vi "Main.vi"() -> ()   [LabVIEW 2018]
doc: "This Continuous Measurement sample project is based on the Queued Message Handler template.\n\nThe Event Handling Loop generates messages based on user interface actions.\n\nThe Message Handling Loop processes messages generated by the Event Handling Loop, or by other messages. There are also Acquisition and Logging message handling loop subVIs, and a chart updating loop."
uses:
  Settings/Settings.ctl
  Acquisition/Hardware Configuration.ctl
  Logging/Logging Configuration.ctl
  controls/UI Data.ctl
  controls/UI State.ctl
  support/Message Queue/Enqueue Message (Single).vi
  support/Message Queue/Enqueue Message (Array).vi
  <vilib>/Utility/error.llb/Error Cluster From Error Code.vi
  <vilib>/ErrorRing/Error Ring.xnode
  Acquisition/Acquisition.lvlib
  Logging/Logging.lvlib
  Settings/Settings.lvlib
  support/User Event - Stop/User Event - Stop.lvlib
  support/Message Queue/Message Queue.lvlib
  Settings/Settings Dialog.vi
panel:
  out "Data":waveform(dbl)[](graph)
  out "Config":T1={"Hardware Configuration"={"DAQmx Channel 1"="SimDev1/ai0", "DAQmx Channel 2"="SimDev1/ai1", "DAQmx Channel 3"="SimDev1/ai2", "Channel 1 Name"="Battery Voltage", "Channel 2 Name"="Battery Current", "Channel 3 Name"="Brake torque", "Input Config Channel 1"=-1, "Input Config Channel 2"=-1, "Input Config Channel 3"=-1, "Offset Channel 1"=0.0, "Offset Channel 2"=0.0, "Offset Channel 3"=0.0, "Scale Channel 1"=0.0, "Scale Channel 2"=0.0, "Scale Channel 3"=0.0, "DAQmx Counter Channel"="", "Counter Name"="", "Sample time"=50, "Samples per second"=1000.0, "Sample mode"=0, "Samples per channel"=0, "DAQmx AI Task"="", "DAQmx Counter Task"=""}, "Logging Configuration"={"Log File Base Path"=path "", "TDMS File Reference"=refnum}} {"Hardware Configuration"."Input Config Channel 3" items=["Default"=-1, "RSE"=10083, "NRSE"=10078, "Differential"=10106, "Pseudodifferential"=12529]; "Hardware Configuration"."Input Config Channel 2" items=["Default"=-1, "RSE"=10083, "NRSE"=10078, "Differential"=10106, "Pseudodifferential"=12529]; "Hardware Configuration"."Input Config Channel 1" items=["Default"=-1, "RSE"=10083, "NRSE"=10078, "Differential"=10106, "Pseudodifferential"=12529]; "Hardware Configuration"."Sample mode" items=["Hardware Timed Single Point"=12522, "Finite Samples"=10178, "Continuous Samples"=10123]}
  in  "Start":bool
  in  "Stop":bool
  in  "Settings":bool
  out "Status":string
  in  "data to matlab":bool
  in  "Exit":bool
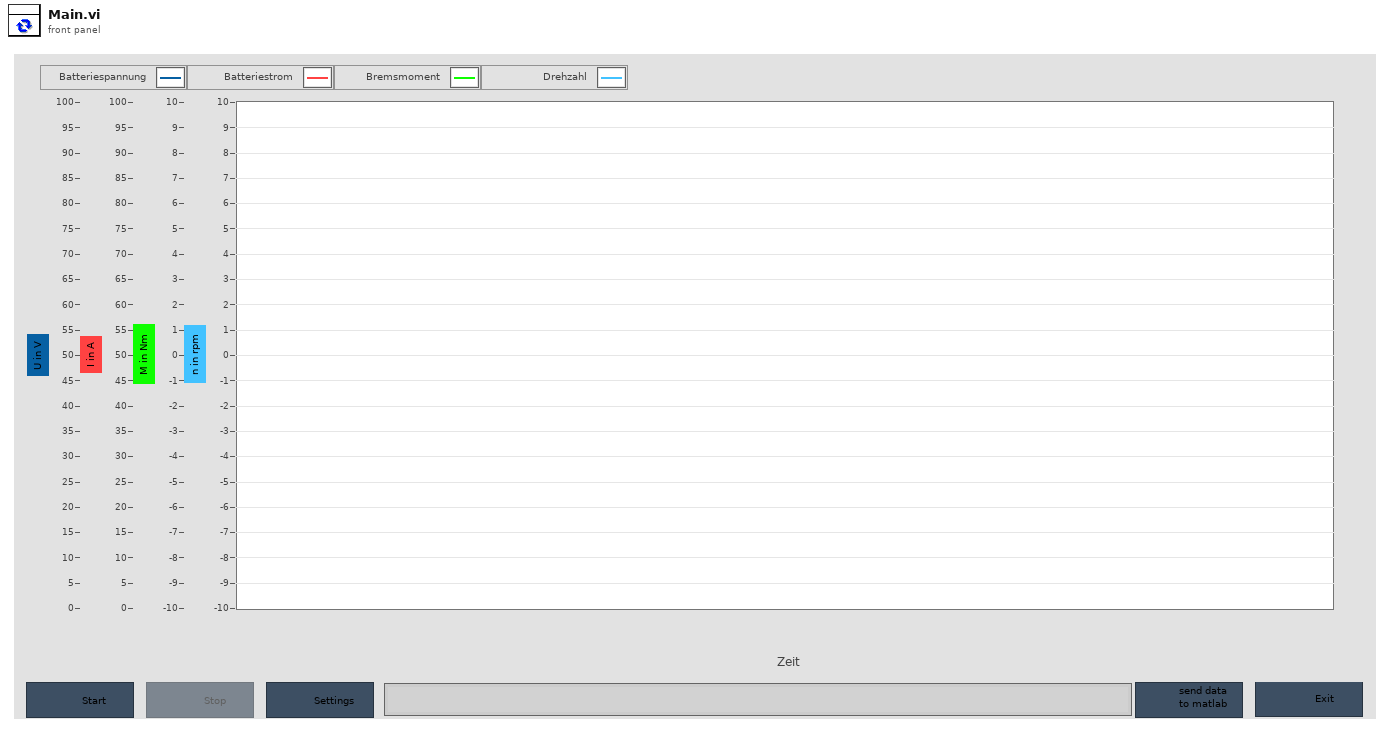
[diagram p1: front panel]
types:
  T1 = typedef "Settings.lvlib/Settings.ctl" = cluster{"Hardware Configuration":T2, "Logging Configuration":T3}
  T2 = typedef "Acquisition.lvlib/Hardware Configuration.ctl" = cluster{"DAQmx Channel 1":tag, "DAQmx Channel 2":tag, "DAQmx Channel 3":tag, "Channel 1 Name":string, "Channel 2 Name":string, "Channel 3 Name":string, "Input Config Channel 1":i32, "Input Config Channel 2":i32, "Input Config Channel 3":i32, "Offset Channel 1":dbl, "Offset Channel 2":dbl, "Offset Channel 3":dbl, "Scale Channel 1":dbl, "Scale Channel 2":dbl, "Scale Channel 3":dbl, "DAQmx Counter Channel":tag, "Counter Name":string, "Sample time":u32, "Samples per second":dbl, "Sample mode":u16, "Samples per channel":i32, "DAQmx AI Task":refnum<k21>, "DAQmx Counter Task":refnum<k21>}
  T3 = typedef "Logging.lvlib/Logging Configuration.ctl" = cluster{"Log File Base Path":path, "TDMS File Reference":refnum<k34>}
  T4 = typedef "UI State.ctl" = enum16{"Idle", "Acquiring and Logging", "Waiting for Exit", "Waiting for Exit (Acq Stopped)", "Waiting for Exit (Log Stopped)", "Waiting for Stop", "Waiting for Stop (Acq Stopped)", "Waiting for Stop (Log Stopped)"}
  T5 = typedef "UI Data.ctl" = cluster{"Start Ref":refnum<vi>, "Stop Ref":refnum<vi>, "Settings Ref":refnum<vi>, "Exit Ref":refnum<vi>, "Status Ref":refnum<vi>, "Data Ref":refnum<vi>, "data to matlab Ref":refnum<vi>}
  T6 = typedef "Message Queue.lvlib/All Message Queues.ctl" = cluster{"UI":refnum<queue>, "Acquisition":refnum<queue>, "Logging":refnum<queue>}
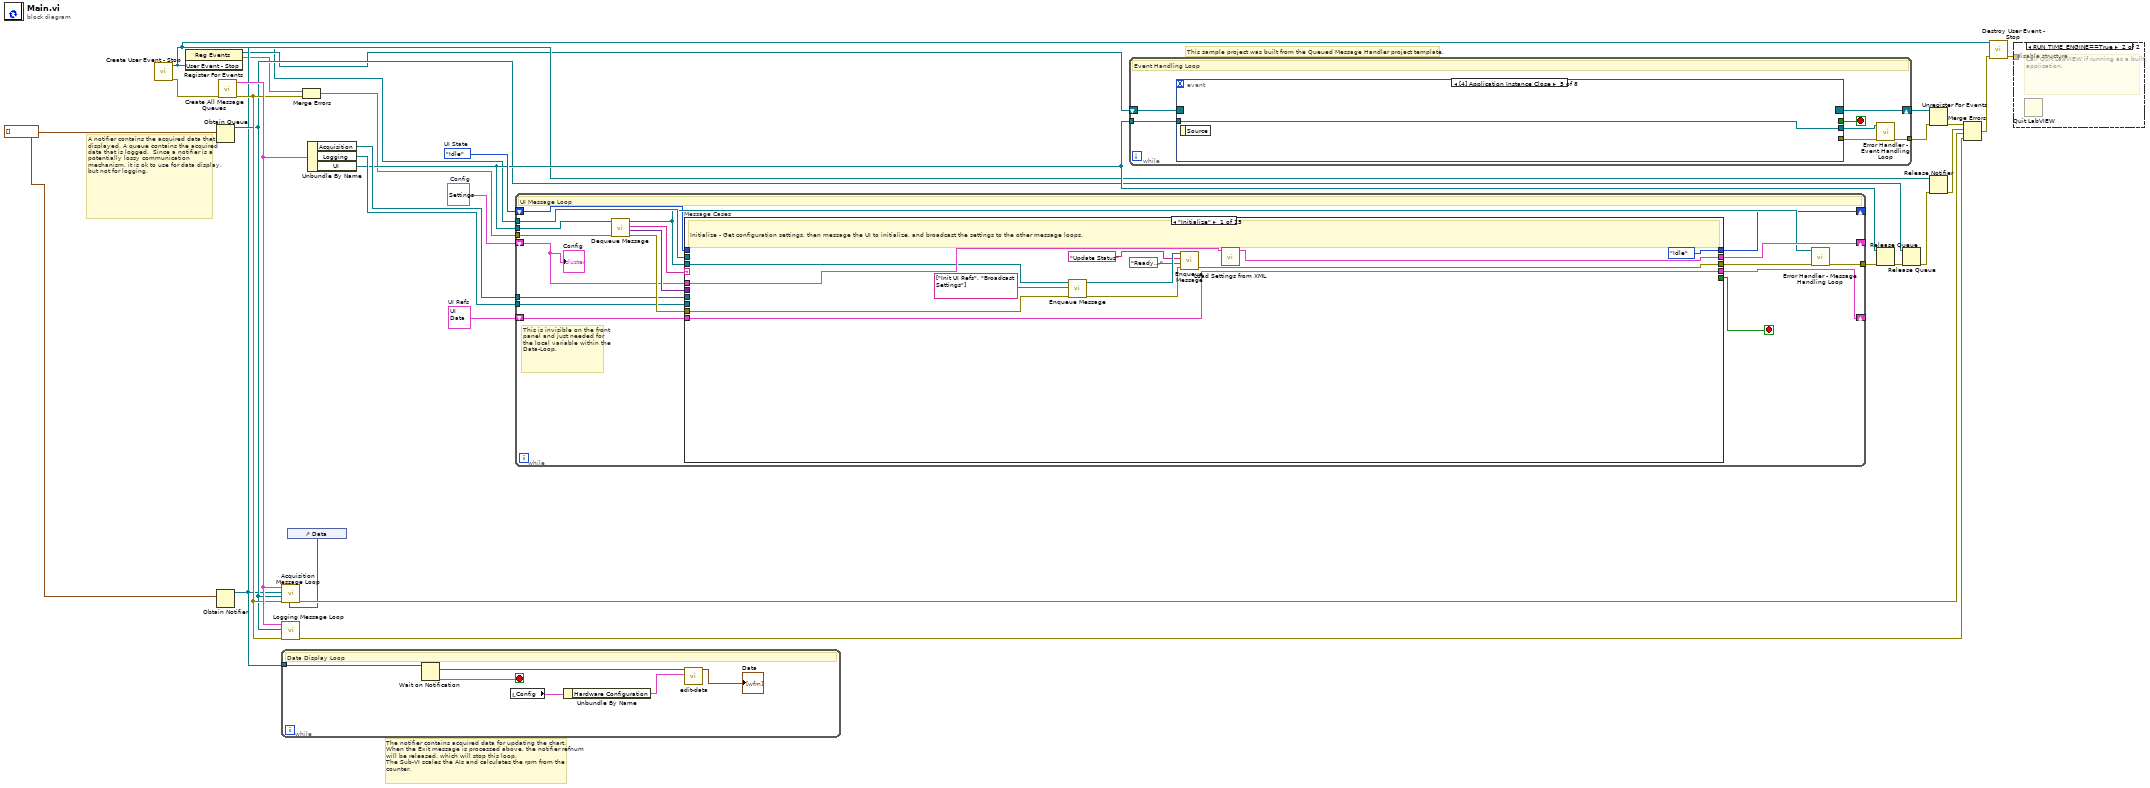
[diagram p0: block diagram]
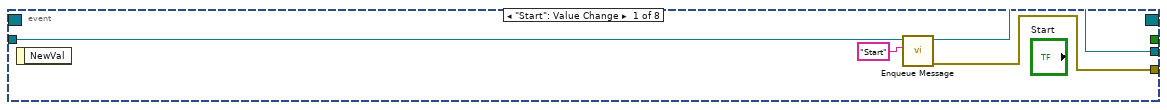
[diagram p3: hidden frame]
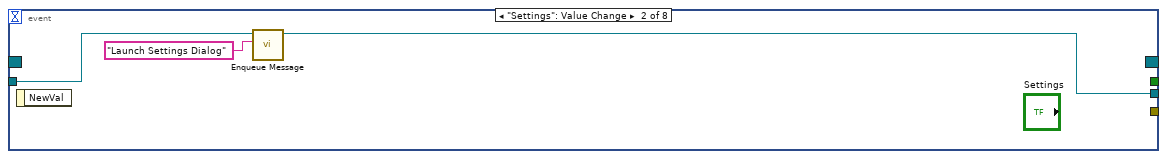
[diagram p4: hidden frame]
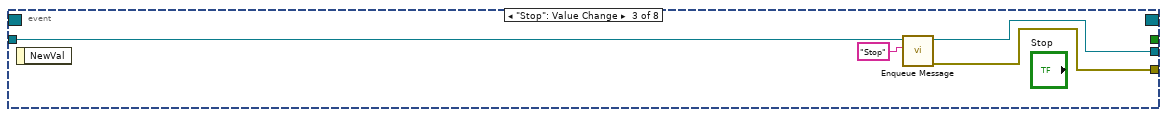
[diagram p5: hidden frame]
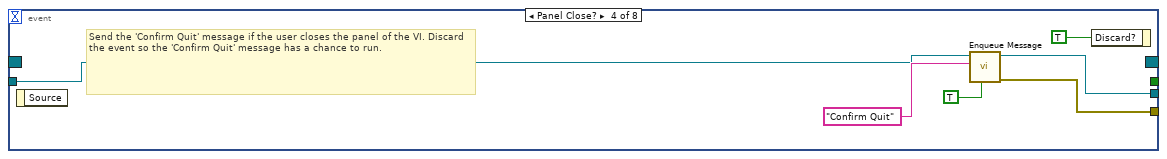
[diagram p6: hidden frame]
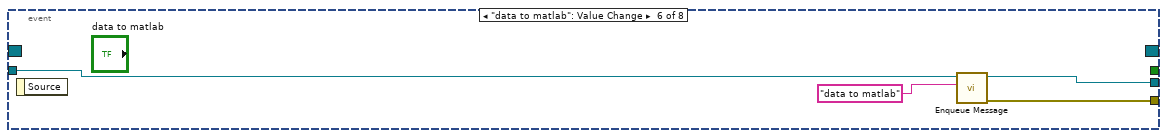
[diagram p7: hidden frame]
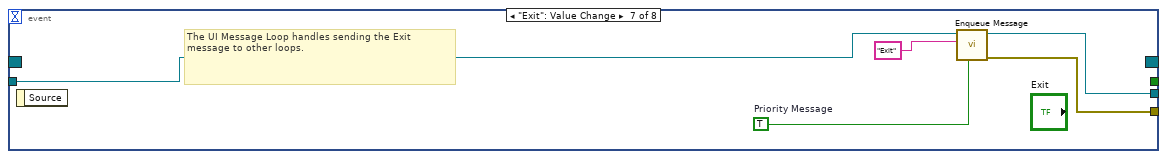
[diagram p8: hidden frame]
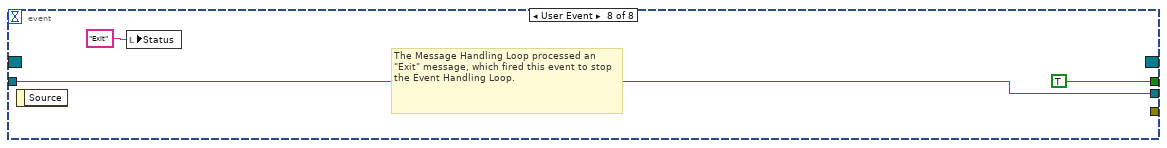
[diagram p9: hidden frame]
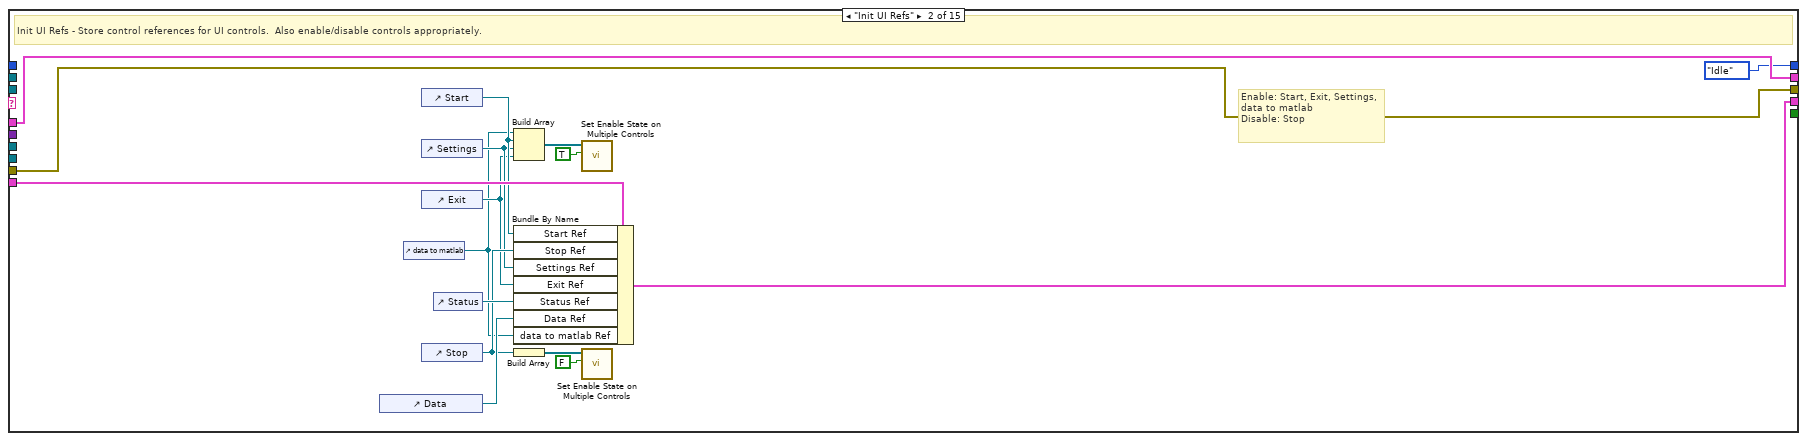
[diagram p10: hidden frame]
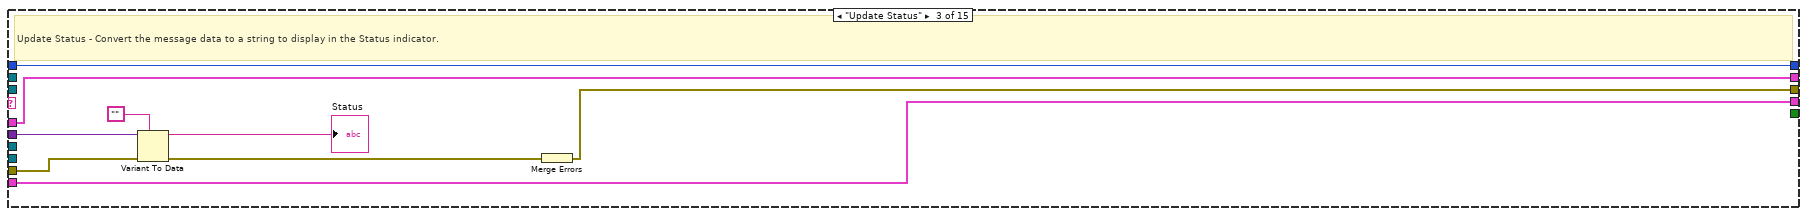
[diagram p11: hidden frame]
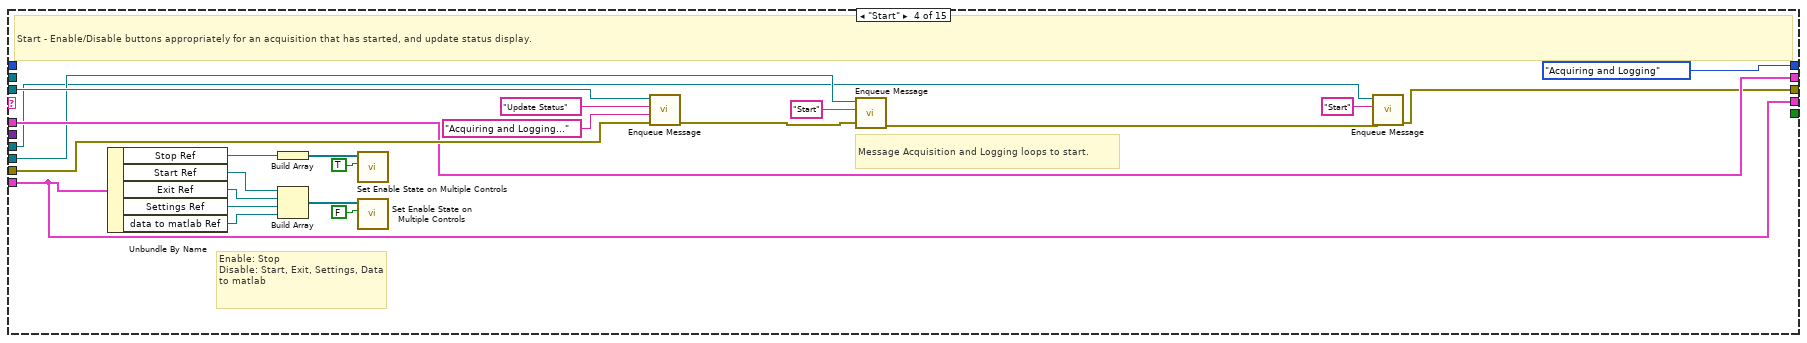
[diagram p12: hidden frame]
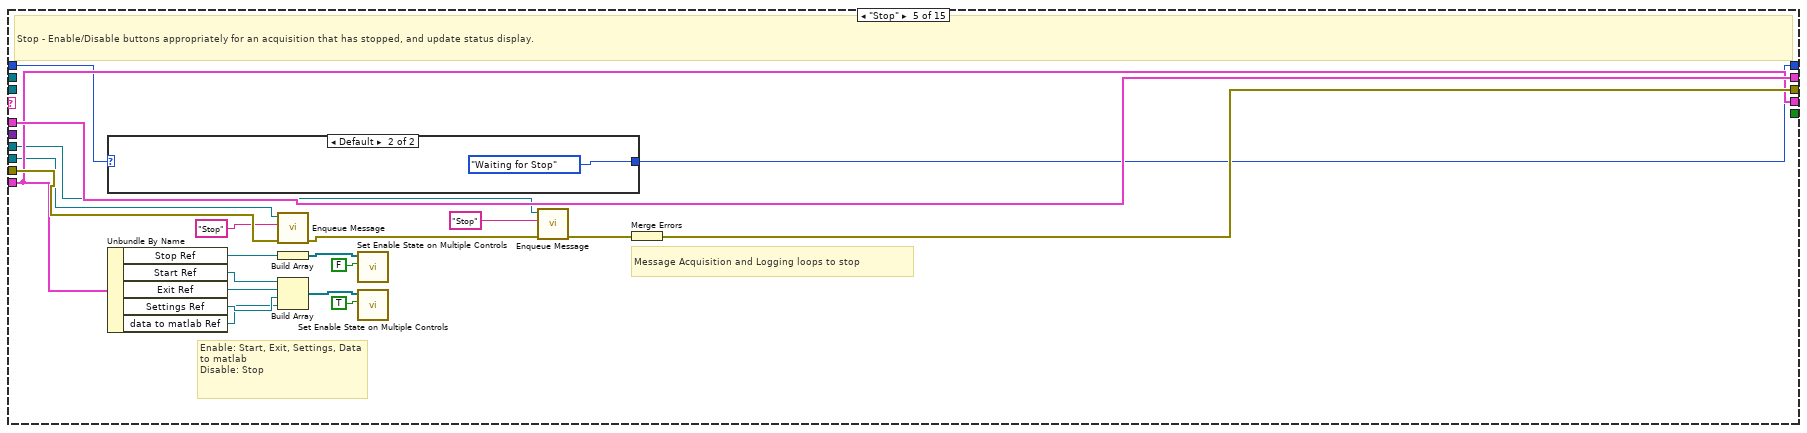
[diagram p13: hidden frame]
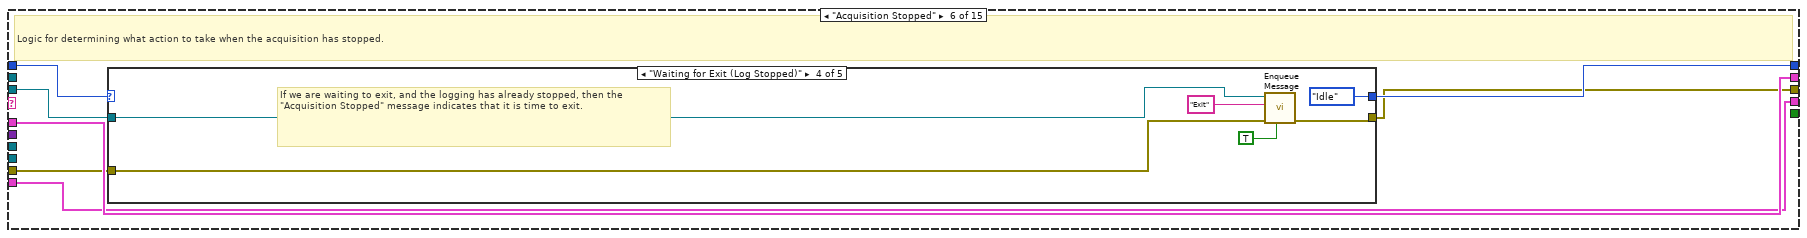
[diagram p15: hidden frame]
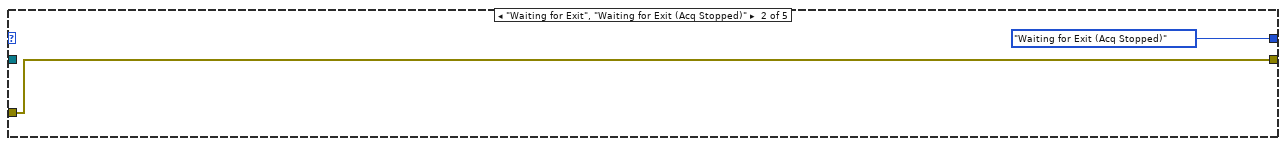
[diagram p17: hidden frame]
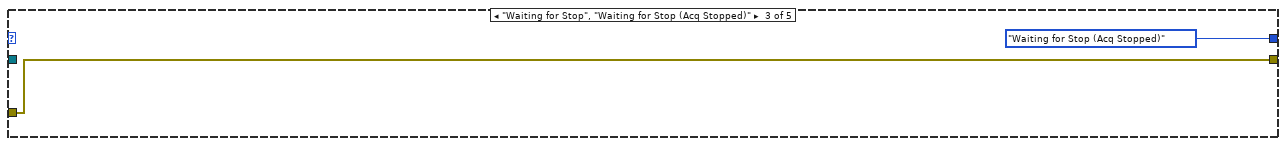
[diagram p18: hidden frame]
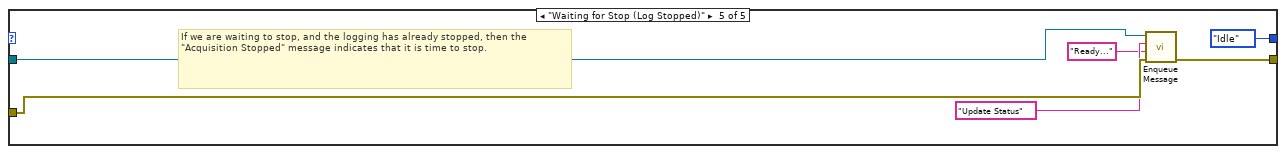
[diagram p19: hidden frame]
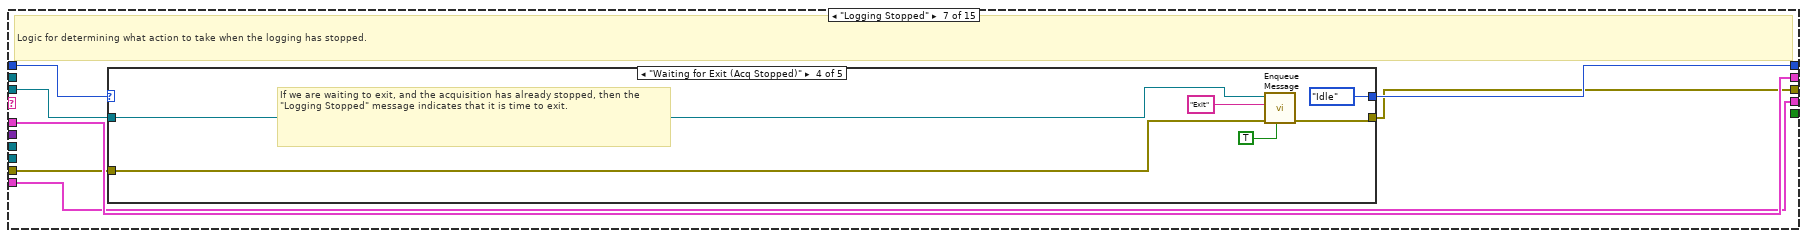
[diagram p20: hidden frame]
diagram:
  w16 = UI_State."Idle"  # UI State
  w7 = waveform(dbl)[] []
  w19 = T5 {"Start Ref"=refnum, "Stop Ref"=refnum, "Settings Ref"=refnum, "Exit Ref"=refnum, "Status Ref"=refnum, "Data Ref"=refnum, "data to matlab Ref"=refnum}  # UI Refs
  w2 = T1 {"Hardware Configuration"={"DAQmx Channel 1"="", "DAQmx Channel 2"="", "DAQmx Channel 3"="", "Channel 1 Name"="Battery Voltage", "Channel 2 Name"="Battery Current", "Channel 3 Name"="Brake torque", "Input Config Channel 1"=-1, "Input Config Channel 2"=-1, "Input Config Channel 3"=-1, "Offset Channel 1"=0.0, "Offset Channel 2"=0.0, "Offset Channel 3"=0.0, "Scale Channel 1"=0.0, "Scale Channel 2"=0.0, "Scale Channel 3"=0.0, "DAQmx Counter Channel"="", "Counter Name"="", "Sample time"=50, "Samples per second"=1000.0, "Sample mode"=0, "Samples per channel"=0, "DAQmx AI Task"="", "DAQmx Counter Task"=""}, "Logging Configuration"={"Log File Base Path"=path "", "TDMS File Reference"=refnum}}  # Config
  # "This sample project was built from the Queued Message Handler project template."
  # "A notifier contains the acquired data that is displayed. A queue contains the acquired data that is logged.  Since a notifier is a potentially lossy communication mechanism, it is ok to use for data display, but not for logging."
  # "The notifier contains acquired data for updating the chart. When the Exit message is processed above, the notifier refnum will be released, which will stop this loop.\nThe Sub-VI scales the AIs and calculates the rpm from the counter."
  n1 = call "Create User Event - Stop.vi"() -> ("error out"=w25:errorcluster, "User Event - Stop"=w5:refnum<user-event>)  [unwired: 10 in]
  n2 = register-events(w5) -> (reference out=w6:refnum<event-registration>, error out=w3:errorcluster)  [unwired: 2 in]
  n3 = Obtain Queue(element data type=w7) -> (queue out=w9:refnum<queue>)  [unwired: 4 in, 2 out]
  n4 = Obtain Notifier(notification data type=w7) -> (notifier out=w8:refnum<notifier>)  [unwired: 3 in, 2 out]
  n5 = call "Create All Message Queues.vi"("error in (no error)"=w25) -> ("error out"=w22:errorcluster, "Message Queues out"=w24:T6)  [unwired: 9 in]
  n6 = call "Logging Message Loop.vi"("error in (no error)"=w22, "Data Queue"=w9, "Message Queues"=w24) -> ("error out"=w23:errorcluster)  [unwired: 8 in]
  n7 = while "Data Display Loop" {
    tunnel: w8 -> [w34]
    stop <- w33 stop-if-true
    # "Data Display Loop"
    n8 = Wait on Notification(notifier=w34) -> (notification=w31:waveform(dbl)[], error out=w33:errorcluster)  [unwired: 3 in, 2 out]
    n9 = local read "Config"() -> (w30:T1)
    n10 = Unbundle By Name(w30) -> ("Hardware Configuration"=w29:T2)
    n11 = call "edit-data.vi"("Hardware Resources in"=w29, "data"=w31) -> ("Array of Waveform"=→"Data":waveform(dbl)[])  [unwired: 9 in]
  }
  n12 = control-ref of="Data"() -> (w1:refnum<vi>)
  n13 = call "Acquisition Message Loop.vi"("Data-Chart-Reference"=w1, "error in (no error)"=w22, "Data Queue"=w9, "Data Notifier"=w8, "Message Queues"=w24) -> ("error out"=w26:errorcluster)  [unwired: 6 in]
  n14 = Merge Errors(w3, w22) -> (w4:errorcluster)
  n15 = Unbundle By Name(w24) -> ("Acquisition"=w18:refnum<queue>, "Logging"=w17:refnum<queue>, "UI"=w14:refnum<queue>)
  n16 = while {
    tunnel: w14 -> [w46]
    tunnel: w5 -> [w51]
    shift-right: [w45] -> _
    shift-left: w2 -> [w35]
    shift-right: [w43] -> _
    shift-left: w19 -> [w44]
    tunnel: w18 -> [w42]
    tunnel: w17 -> [w41]
    shift-right: [w36] -> _
    shift-left: w16 -> [w37]
    tunnel: w4 -> [w50]
    tunnel: [w40] -> w28
    stop <- w52 stop-if-true
    # "This is invisible on the front panel and just needed for the local variable within the Data-Loop."
    # "UI Message Loop"
    n17 = call "Dequeue Message.vi"("error in (no error)"=w50, "Message Queue"=w46) -> ("error out"=w49:errorcluster, "Message Data"=w47:variant, "Message"=w48:string, "dup Message Queue"=w38:refnum<queue>)  [unwired: 6 in]
    n18 = case "Message Cases" shown="\"Initialize\"" w48 {
      selector: w48 -> [_ _ _ _ _ _ _ _ _ _ _ _ _ _ w277]
      tunnel: w38 -> [w56 _ _ w112 _ w138 w163 _ w203 _ w224 _ _ _ _]
      tunnel: w49 -> [w55 w80 w88 w111 w132 w139 w164 w191 w205 w212 w223 w252 w269 w275 _]
      tunnel: [w60 w80 w89 w94 w133 w136 w161 w197 w198 w215 w222 w262 w268 w270 w276] -> w39
      tunnel: [_ _ _ _ _ _ _ _ _ _ _ TRUE _ _ _] -> w52
      tunnel: w47 -> [_ _ w87 _ _ _ _ _ _ w216 _ w250 _ _ _]
      tunnel: w51 -> [_ _ _ _ _ _ _ _ _ _ _ w263 _ _ _]
      tunnel: [w63 w79 w83 w110 w131 w142 w167 w195 w202 w220 w227 w261 w267 w272 w280] -> w45
      tunnel: w35 -> [w64 w79 w83 w110 w131 w142 w167 w195 w206 w220 w227 w261 w267 w272 w280]
      tunnel: w44 -> [w57 w78 w82 w107 w130 w141 w166 w189 w200 w219 w226 w260 w266 w274 w279]
      tunnel: [w57 w75 w82 w107 w130 w141 w166 w189 w200 w219 w226 w260 w266 w274 w279] -> w43
      tunnel: w42 -> [_ _ _ w93 w117 _ _ w188 _ _ _ w259 _ _ _]
      tunnel: w41 -> [_ _ _ w96 w120 _ _ w187 _ _ _ w258 _ _ _]
      tunnel: w37 -> [_ _ w81 _ w114 w140 w165 w186 w199 w214 w225 _ w265 w273 w278]
      tunnel: [UI_State."Idle" ("UI State") UI_State."Idle" ("UI State") w81 UI_State."Acquiring and Logging" ("UI State") w115 w137 w162 w186 w199 w214 w221 UI_State."Idle" ("UI State") w265 w273 w278] -> w36
      frame "Initialize" {
        # "Initialize - Get configuration settings, then message the UI to initialize, and broadcast the settings to the other message loops."
        n19 = call-poly "Enqueue Message.vi"("error in (no error)"=w55, "Message Array"=string[] ["Init UI Refs", "Broadcast Settings"], "Message Queue"=w56) -> ("error out"=w62:errorcluster, "dup Message Queue"=w61:refnum<queue>)  [unwired: 7 in]
        n20 = call-poly "Enqueue Message.vi"("error in (no error)"=w62, "Message Data"="Ready..." ("Ready..."), "Message"="Update Status", "Message Queue"=w61) -> ("error out"=w60:errorcluster)  [unwired: 6 in, 1 out]
        n21 = call "Load Settings from XML.vi"("Settings in"=w64) -> ("Settings out"=w63:T1)  [unwired: 9 in, 1 out]
      }
      frame "Init UI Refs" {
        # "Enable: Start, Exit, Settings, data to matlab\nDisable: Stop"
        # "Init UI Refs - Store control references for UI controls.  Also enable/disable controls appropriately."
        n22 = control-ref of="Data"() -> (w76:refnum<vi>)
        n23 = control-ref of="data to matlab"() -> (w65:refnum<vi>)
        n24 = control-ref of="Start"() -> (w69:refnum<vi>)
        n25 = control-ref of="Settings"() -> (w68:refnum<vi>)
        n26 = control-ref of="Exit"() -> (w67:refnum<vi>)
        n27 = control-ref of="Stop"() -> (w70:refnum<vi>)
        n28 = control-ref of="Status"() -> (w77:refnum<vi>)
        n29 = Build Array(w65, w69, w68, w67) -> (w73:refnum<vi>[])
        n30 = Bundle By Name(cluster=w78, "Start Ref"=w69, "Stop Ref"=w70, "Settings Ref"=w68, "Exit Ref"=w67, "Status Ref"=w77, "Data Ref"=w76, "data to matlab Ref"=w65) -> (w75:T5)
        n31 = Build Array(w70) -> (w72:refnum<vi>[])
        n32 = call "Set Enable State on Multiple Controls.vi"("Enable?"=TRUE, "Controls"=w73) -> ()  [unwired: 10 in]
        n33 = call "Set Enable State on Multiple Controls.vi"("Enable?"=FALSE, "Controls"=w72) -> ()  [unwired: 10 in]
      }
      frame "Update Status" {
        # "Update Status - Convert the message data to a string to display in the Status indicator."
        n34 = Variant To Data(error in=w88, type="", Variant=w87) -> (data=→"Status":string, error out=w85:errorcluster)
        n35 = Merge Errors(w85) -> (w89:errorcluster)
      }
      frame "Start" {
        # "Message Acquisition and Logging loops to start."
        # "Enable: Stop\nDisable: Start, Exit, Settings, Data to matlab"
        # "Start - Enable/Disable buttons appropriately for an acquisition that has started, and update status display."
        n36 = Unbundle By Name(w107) -> ("Stop Ref"=w102:refnum<vi>, "Start Ref"=w101:refnum<vi>, "Exit Ref"=w100:refnum<vi>, "Settings Ref"=w99:refnum<vi>, "data to matlab Ref"=w90:refnum<vi>)
        n37 = Build Array(w102) -> (w104:refnum<vi>[])
        n38 = Build Array(w101, w100, w99, w90) -> (w105:refnum<vi>[])
        n39 = call "Set Enable State on Multiple Controls.vi"("Enable?"=TRUE, "Controls"=w104) -> ()  [unwired: 10 in]
        n40 = call "Set Enable State on Multiple Controls.vi"("Enable?"=FALSE, "Controls"=w105) -> ()  [unwired: 10 in]
        n41 = call-poly "Enqueue Message.vi"("error in (no error)"=w111, "Message Data"="Acquiring and Logging..." ("Acquiring and Logging..."), "Message"="Update Status", "Message Queue"=w112) -> ("error out"=w98:errorcluster)  [unwired: 6 in, 1 out]
        n42 = call-poly "Enqueue Message.vi"("error in (no error)"=w98, "Message"="Start", "Message Queue"=w96) -> ("error out"=w95:errorcluster)  [unwired: 7 in, 1 out]
        n43 = call-poly "Enqueue Message.vi"("error in (no error)"=w95, "Message"="Start", "Message Queue"=w93) -> ("error out"=w94:errorcluster)  [unwired: 7 in, 1 out]
      }
      frame "Stop" {
        # "Message Acquisition and Logging loops to stop"
        # "Enable: Start, Exit, Settings, Data to matlab\nDisable: Stop"
        # "Stop - Enable/Disable buttons appropriately for an acquisition that has stopped, and update status display."
        n44 = case shown="Default" w114 {
          selector: w114 -> [w134 _]
          tunnel: [w134 UI_State."Waiting for Stop" ("UI State")] -> w115
          frame "Waiting for Exit" {
          }
          frame Default {
          }
        }
        n45 = Unbundle By Name(w130) -> ("Stop Ref"=w125:refnum<vi>, "Start Ref"=w124:refnum<vi>, "Exit Ref"=w123:refnum<vi>, "Settings Ref"=w122:refnum<vi>, "data to matlab Ref"=w113:refnum<vi>)
        n46 = call-poly "Enqueue Message.vi"("error in (no error)"=w132, "Message"="Stop", "Message Queue"=w120) -> ("error out"=w119:errorcluster)  [unwired: 7 in, 1 out]
        n47 = Build Array(w125) -> (w127:refnum<vi>[])
        n48 = Build Array(w124, w123, w122, w113) -> (w128:refnum<vi>[])
        n49 = call "Set Enable State on Multiple Controls.vi"("Enable?"=FALSE, "Controls"=w127) -> ()  [unwired: 10 in]
        n50 = call "Set Enable State on Multiple Controls.vi"("Enable?"=TRUE, "Controls"=w128) -> ()  [unwired: 10 in]
        n51 = call-poly "Enqueue Message.vi"("error in (no error)"=w119, "Message"="Stop", "Message Queue"=w117) -> ("error out"=w118:errorcluster)  [unwired: 7 in, 1 out]
        n52 = Merge Errors(w118) -> (w133:errorcluster)
      }
      frame "Acquisition Stopped" {
        # "Logic for determining what action to take when the acquisition has stopped."
        n53 = case shown="\"Waiting for Exit (Log Stopped)\"" w140 {
          selector: w140 -> [w144 _ _ _ _]
          tunnel: w139 -> [w143 w146 w148 w154 w160]
          tunnel: w138 -> [_ _ _ w152 w157]
          tunnel: [w144 UI_State."Waiting for Exit (Acq Stopped)" ("UI State") UI_State."Waiting for Stop (Acq Stopped)" ("UI State") UI_State."Idle" ("UI State") UI_State."Idle" ("UI State")] -> w137
          tunnel: [w143 w146 w148 w153 w158] -> w136
          frame Default {
          }
          frame "Waiting for Exit", "Waiting for Exit (Acq Stopped)" {
          }
          frame "Waiting for Stop", "Waiting for Stop (Acq Stopped)" {
          }
          frame "Waiting for Exit (Log Stopped)" {
            # "If we are waiting to exit, and the logging has already stopped, then the \"Acquisition Stopped\" message indicates that it is time to exit."
            n54 = call-poly "Enqueue Message.vi"("Priority Message? (F)"=TRUE, "error in (no error)"=w154, "Message"="Exit", "Message Queue"=w152) -> ("error out"=w153:errorcluster)  [unwired: 6 in, 1 out]
          }
          frame "Waiting for Stop (Log Stopped)" {
            # "If we are waiting to stop, and the logging has already stopped, then the \"Acquisition Stopped\" message indicates that it is time to stop."
            n55 = call-poly "Enqueue Message.vi"("error in (no error)"=w160, "Message Data"="Ready..." ("Ready..."), "Message"="Update Status", "Message Queue"=w157) -> ("error out"=w158:errorcluster)  [unwired: 6 in, 1 out]
          }
        }
      }
      frame "Logging Stopped" {
        # "Logic for determining what action to take when the logging has stopped."
        n56 = case shown="\"Waiting for Exit (Acq Stopped)\"" w165 {
          selector: w165 -> [w169 _ _ _ _]
          tunnel: w164 -> [w168 w171 w173 w179 w182]
          tunnel: w163 -> [_ _ _ w177 w181]
          tunnel: [w169 UI_State."Waiting for Exit (Log Stopped)" ("UI State") UI_State."Waiting for Stop (Log Stopped)" ("UI State") UI_State."Idle" ("UI State") UI_State."Idle" ("UI State")] -> w162
          tunnel: [w168 w171 w173 w178 w180] -> w161
          frame Default {
          }
          frame "Waiting for Exit", "Waiting for Exit (Log Stopped)" {
          }
          frame "Waiting for Stop", "Waiting for Stop (Log Stopped)" {
          }
          frame "Waiting for Exit (Acq Stopped)" {
            # "If we are waiting to exit, and the acquisition has already stopped, then the \"Logging Stopped\" message indicates that it is time to exit."
            n57 = call-poly "Enqueue Message.vi"("Priority Message? (F)"=TRUE, "error in (no error)"=w179, "Message"="Exit", "Message Queue"=w177) -> ("error out"=w178:errorcluster)  [unwired: 6 in, 1 out]
          }
          frame "Waiting for Stop (Acq Stopped)" {
            # "If we are waiting to stop, and the acquisition has already stopped, then the \"Logging Stopped\" message indicates that it is time to stop."
            n58 = call-poly "Enqueue Message.vi"("error in (no error)"=w182, "Message Data"="Ready..." ("Ready..."), "Message"="Update Status", "Message Queue"=w181) -> ("error out"=w180:errorcluster)  [unwired: 6 in, 1 out]
          }
        }
      }
      frame "Broadcast settings" {
        w190 = "Update Settings" ("Message")
        # "Broadcast settings - Send the 'Update Settings' message to the Logging and Acquisition message loops."
        n59 = Unbundle By Name(w195) -> ("Hardware Configuration"=w194:T2, "Logging Configuration"=w193:T3)
        n60 = call-poly "Enqueue Message.vi"("Message Data"=w194, "Message"=w190, "Message Queue"=w188) -> ("error out"=w196:errorcluster)  [unwired: 7 in, 1 out]
        n61 = call-poly "Enqueue Message.vi"("error in (no error)"=w196, "Message Data"=w193, "Message"=w190, "Message Queue"=w187) -> ("error out"=w192:errorcluster)  [unwired: 6 in, 1 out]
        n62 = Merge Errors(w192, w191) -> (w197:errorcluster)
      }
      frame "Launch Settings Dialog" {
        # "Launch Settings Dialog - Launch the Settings Dialog when the user clicks the 'Settings' button."
        n63 = call-by-ref "?"("error in (no error)"=w205, "Settings in"=w206) -> ("error out"=w201:errorcluster, "Cancelled?"=w204:bool, "Settings out"=w202:T1)  [unwired: 8 in, 3 out]
        n64 = case shown="False" w204 {
          tunnel: w203 -> [w210 _]
          tunnel: w201 -> [w209 w211]
          tunnel: [w208 w211] -> w198
          frame False {
            n65 = call-poly "Enqueue Message.vi"("error in (no error)"=w209, "Message"="Broadcast Settings", "Message Queue"=w210) -> ("error out"=w208:errorcluster)  [unwired: 7 in, 1 out]
          }
          frame True {
          }
        }
      }
      frame "Error" {
        # "Error - Display an error dialog. This message is sent by the \"Error Handler\" VIs at the end of other loops in this application."
        n66 = Variant To Data(error in=w212, type=errorcluster {"status"=FALSE, "code"=0, "source"=""} ("error constant"), Variant=w216) -> (data=w213:errorcluster, error out=w217:errorcluster)
        n67 = call <vilib>:"Simple Error Handler.vi"("error in (no error)"=w213) -> ()  [unwired: 4 in, 5 out]
        n68 = Merge Errors(w217) -> (w215:errorcluster)
      }
      frame "Confirm Quit" {
        # "Confirm Quit - Message that can confirm whether or not the user wants to exit the application."
        n69 = case shown="\"Acquiring and Logging\"" w225 {
          tunnel: w224 -> [w233 w237]
          tunnel: w223 -> [w232 w236]
          tunnel: [w231 w235] -> w222
          tunnel: [UI_State."Idle" ("UI State") w234] -> w221
          frame Default {
            # "If 'Confirm Quit' comes in while the system is idle, there is no need for a confirmation message."
            n70 = call-poly "Enqueue Message.vi"("Priority Message? (F)"=TRUE, "error in (no error)"=w232, "Message"="Exit", "Message Queue"=w233) -> ("error out"=w231:errorcluster)  [unwired: 6 in, 1 out]
          }
          frame "Acquiring and Logging" {
            n71 = Two Button Dialog(message="Are you sure you want to quit while the acquisition is running?" ("Confirm Quit Message"), 1:"No" ("No"), 2:"Yes" ("Yes")) -> (T button?=w238:bool)
            n72 = case shown="True" w238 {
              tunnel: w237 -> [_ w247]
              tunnel: w236 -> [w243 w248]
              tunnel: [w243 w246] -> w235
              tunnel: [UI_State."Acquiring and Logging" ("UI State") UI_State."Waiting for Exit" ("UI State")] -> w234
              frame False {
                # "User did not want to quit."
              }
              frame True {
                n73 = call-poly "Enqueue Message.vi"("error in (no error)"=w248, "Message"="Stop", "Message Queue"=w247) -> ("error out"=w246:errorcluster)  [unwired: 7 in, 1 out]
              }
            }
          }
        }
      }
      frame "Exit" {
        w254 = TRUE ("Priority Message? (F)")
        w255 = "Exit" ("Message")
        # "Popup an error dialog if 'Exit' was called as a result of an error."
        # "Stop the VI"
        # "Exit - Send Exit messages to the Acquisition and Logging loops, and fire the user event to stop the Event Handling Loop."
        n74 = Variant To Data(type=errorcluster {"status"=FALSE, "code"=0, "source"=""} ("error constant"), Variant=w250) -> (data=w249:errorcluster)  [unwired: 1 in, 1 out]
        n75 = call-poly "Enqueue Message.vi"("Priority Message? (F)"=w254, "error in (no error)"=w252, "Message"=w255, "Message Queue"=w259) -> ("error out"=w256:errorcluster)  [unwired: 6 in, 1 out]
        n76 = call <vilib>:"Simple Error Handler.vi"("error in (no error)"=w249) -> ()  [unwired: 4 in, 5 out]
        n77 = call-poly "Enqueue Message.vi"("Priority Message? (F)"=w254, "error in (no error)"=w256, "Message"=w255, "Message Queue"=w258) -> ("error out"=w253:errorcluster)  [unwired: 6 in, 1 out]
        n78 = call "Fire User Event - Stop.vi"("error in (no error)"=w253, "User Event - Stop"=w263) -> ("error out"=w262:errorcluster)  [unwired: 9 in]
      }
      frame "---Copy This Frame---" {
        # "Duplicate this frame when creating new messages.  Change this comment in the duplicated frame to describe this message."
        n79 = Merge Errors(w269) -> (w268:errorcluster)
      }
      frame "data to matlab" {
        # "reads the tdms-file from settings, splits the signal into inputs and time, converts the timearray to relative time and forwards the variables to matlab for further inspection"
        n80 = Merge Errors(w275) -> (w271:errorcluster)
        n81 = call "data-to-matlab.vi"("error in (no error)"=w271, "Config"=w272) -> ("error out"=w270:errorcluster)  [unwired: 9 in]
      }
      frame Default {
        # "'Default' case only runs if there is a message that isn't defined in any of the other cases.  Output a programming error."
        n82 = xnode "Error Ring"("parameter 0"=w277) -> ("error out"=w276:errorcluster)
      }
    }
    n83 = call "Error Handler - Message Handling Loop.vi"("error in (no error)"=w39, "Message Queue"=w38) -> ("dup error in"=w40:errorcluster)  [unwired: 8 in, 1 out]
    "Config" <- w35
  }
  n84 = while {
    tunnel: w14 -> [w293]
    tunnel: [w290] -> w27
    shift-right: [w292] -> w20
    shift-left: w6 -> [w294]
    stop <- w291 stop-if-true
    # "Event Handling Loop"
    n85 = event shown="[4] Application Instance Close" {
      selector: w294 -> [_ _ _ _ _ _ _ _]
      dyn-events: [_ _ _ _ _ _ _ _] -> w292
      timeout: _ -> [_ _ _ _ _ _ _ _]
      tunnel: [_ _ _ _ _ _ _ TRUE ("Discard?")] -> w291
      tunnel: w293 -> [w298 w300 w304 w309 w312 w316 w318 w322]
      tunnel: [w296 _ w303 w307 _ w314 w321 _] -> w289
      tunnel: [w295 w299 w302 w308 w312 w315 w317 w322] -> w288
      event "Start": Value Change {
        n86 = event-data() -> ()  [unwired: 1 in, 1 out]
        n87 = call-poly "Enqueue Message.vi"("Message"="Start", "Message Queue"=w298) -> ("error out"=w296:errorcluster, "dup Message Queue"=w295:refnum<queue>)  [unwired: 8 in]
      }
      event "Settings": Value Change {
        n88 = event-data() -> ()  [unwired: 1 in, 1 out]
        n89 = call-poly "Enqueue Message.vi"("Message"="Launch Settings Dialog", "Message Queue"=w300) -> ("dup Message Queue"=w299:refnum<queue>)  [unwired: 8 in, 1 out]
      }
      event "Stop": Value Change {
        n90 = event-data() -> ()  [unwired: 1 in, 1 out]
        n91 = call-poly "Enqueue Message.vi"("Message"="Stop", "Message Queue"=w304) -> ("error out"=w303:errorcluster, "dup Message Queue"=w302:refnum<queue>)  [unwired: 8 in]
      }
      event Panel Close? {
        # "Send the 'Confirm Quit' message if the user closes the panel of the VI. Discard the event so the 'Confirm Quit' message has a chance to run."
        n92 = event-data() -> ()  [unwired: 1 in, 1 out]
        n93 = call-poly "Enqueue Message.vi"("Priority Message? (F)"=TRUE, "Message"="Confirm Quit", "Message Queue"=w309) -> ("error out"=w307:errorcluster, "dup Message Queue"=w308:refnum<queue>)  [unwired: 7 in]
        n94 = event-data("Discard?"=TRUE) -> ()  [unwired: 1 in, 1 out]
      }
      event Application Instance Close {
        n95 = event-data() -> ()  [unwired: 1 in, 1 out]
      }
      event "data to matlab": Value Change {
        n96 = event-data() -> ()  [unwired: 1 in, 1 out]
        n97 = call-poly "Enqueue Message.vi"("Message"="data to matlab", "Message Queue"=w316) -> ("error out"=w314:errorcluster, "dup Message Queue"=w315:refnum<queue>)  [unwired: 8 in]
      }
      event "Exit": Value Change {
        w319 = TRUE  # Priority Message
        # "The UI Message Loop handles sending the Exit message to other loops."
        n98 = event-data() -> ()  [unwired: 1 in, 1 out]
        n99 = call-poly "Enqueue Message.vi"("Priority Message? (F)"=w319, "Message"="Exit", "Message Queue"=w318) -> ("error out"=w321:errorcluster, "dup Message Queue"=w317:refnum<queue>)  [unwired: 7 in]
      }
      event User Event {
        # "The Message Handling Loop processed an \"Exit\" message, which fired this event to stop the Event Handling Loop."
        n100 = event-data() -> ()  [unwired: 1 in, 1 out]
        n101 = local write "Status"("Exit" ("Exit String")) -> ()
      }
    }
    n102 = call "Error Handler - Event Handling Loop.vi"("error in (no error)"=w289, "Message Queue"=w288) -> ("dup error in"=w290:errorcluster)  [unwired: 8 in, 1 out]
  }
  n103 = Release Queue(queue=w14, error in (no error)=w28) -> (error out=w12:errorcluster)  [unwired: 1 in, 2 out]
  n104 = Release Queue(queue=w9, error in (no error)=w12) -> (error out=w11:errorcluster)  [unwired: 1 in, 2 out]
  n105 = Unregister For Events(event registration refnum=w20, error in=w27) -> (error out=w21:errorcluster)
  n106 = Release Notifier(notifier=w8, error in (no error)=w11) -> (error out=w10:errorcluster)  [unwired: 1 in, 2 out]
  n107 = Merge Errors(w21, w10, w26, w23) -> (w15:errorcluster)
  n108 = call "Destroy User Event - Stop.vi"("error in (no error)"=w15, "User Event - Stop"=w5) -> ("error out"=w13:errorcluster)  [unwired: 9 in]
  n109 = disable-structure shown="RUN_TIME_ENGINE==True" {
    disable-tunnel: w13 -> [_ _]
    frame condition #0 (active) {
    }
    frame condition #1 {
      # "Call Quit LabVIEW if running as a built application."
      n110 = Quit LabVIEW() -> ()  [unwired: 1 in]
    }
  }
